vi "Grey Out PNG Image.vi"(8 "error in (no error)":errorcluster, 11 "Image Data in":T1) -> (0 "error out":errorcluster, 3 "Image Data out":T1)   [LabVIEW 2013]
doc: "This VI will take <B>Image Data in</B> and create <B>Image Data out</B> which is the same image with 50% transparency from the original. This will make the image appear greyed out or disabled. Note that this function only works with images that have opacity in the image data like 32Bit images. If the image data is not 32Bit it will be converted to it with the assumption that all pixels are solid.\n\n-----\nBrian Hoover (hooovahh)"
uses:
  <vilib>/picture/picture.llb/imagedata.ctl
  <vilib>/Utility/colorconv.llb/Color to RGB.vi
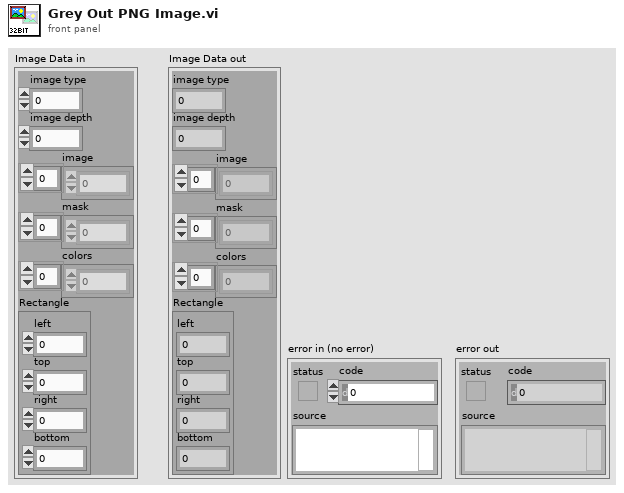
[diagram p1: front panel]
types:
  T1 = typedef "imagedata.ctl" = cluster{"image type":i32, "image depth":i32, "image":u8[], "mask":u8[], "colors":u32[], "Rectangle":cluster{"left":i16, "top":i16, "right":i16, "bottom":i16}}
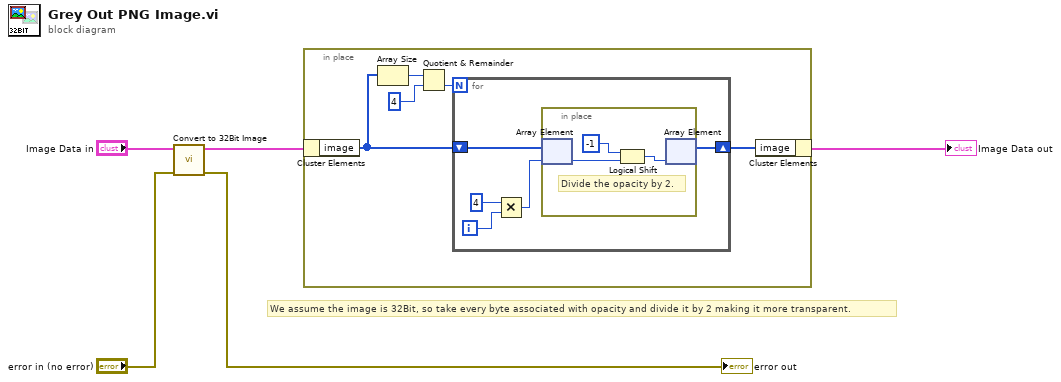
[diagram p0: block diagram]
diagram:
  # "We assume the image is 32Bit, so take every byte associated with opacity and divide it by 2 making it more transparent."
  n1 = call "Convert to 32Bit Image.vi"("error in (no error)"="error in (no error)", "Image Data"="Image Data in") -> ("error out"=→"error out":errorcluster, "32Bit Image Data Out"=w3:T1)  [unwired: 8 in]
  n2 = in-place {
    n3 = in-place-cluster #1(w3) -> ("image"=w7:u8[])
    n4 = Array Size(array=w7) -> (size(s)=w8:i32)
    n5 = Quotient & Remainder(x=w8, y=4) -> (floor(x/y)=w6:i32)  [unwired: 1 out]
    n6 = for {
      N: w6 -> [_]
      shift-right: [w14] -> w10
      shift-left: w7 -> [w15]
      i -> [w12]
      n7 = Multiply(x=4, y=w12) -> (x*y=w11:i32)
      n8 = in-place {
        # "Divide the opacity by 2."
        n9 = in-place-array #2(w15, w11) -> (w17:u8)
        n10 = Logical Shift(y=i8 -1, x=w17) -> (x << y=w16:u8)
        n11 = in-place-array #2(w16) -> (w14:u8[])  [unwired: 1 out]
      }
    }
    n12 = in-place-cluster #1("image"=w10) -> (→"Image Data out":T1)
  }
